vi "SetVariables.vi"(9 "Dynamic Runtime Property Vaslue":string, 10 "Dynamic Property Value":string, 11 "Sequence Context In":refnum<k7>) -> (0 "error out":errorcluster)   [LabVIEW 2011]
doc: "This VI demonstrates how to cast a SequenceFile object in order access properties of the PropertyObjectFile and PropertyObject parent classes"
uses:
  <vilib>/addons/TestStand/_TSUtility.llb/TestStand - Set Property Value (String).vi
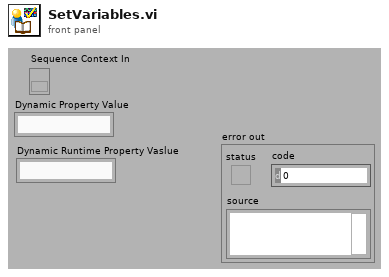
[diagram p1: front panel]
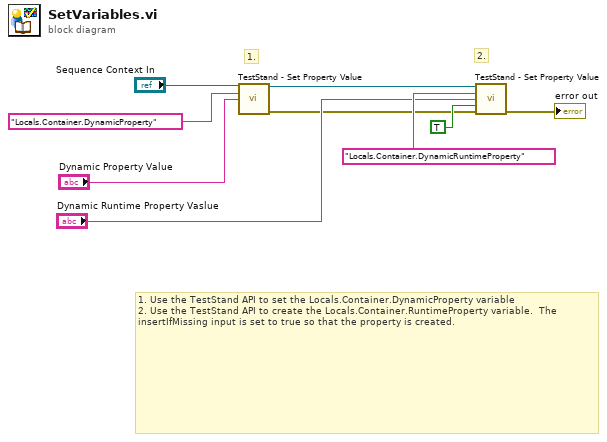
[diagram p0: block diagram]
diagram:
  # "2."
  # "1."
  # "1. Use the TestStand API to set the Locals.Container.DynamicProperty variable\n2. Use the TestStand API to create the Locals.Container.RuntimeProperty variable.  The insertIfMissing input is set to true so that the property is created."
  n1 = call-poly <vilib>:"TestStand - Set Property Value.vi"("Sequence Context In"="Sequence Context In", "Lookup String"="Locals.Container.DynamicProperty", "New Value"="Dynamic Property Value") -> ("Sequence Context Out"=w2:refnum<k7>, "error out"=w3:errorcluster)  [unwired: 11 in]
  n2 = call-poly <vilib>:"TestStand - Set Property Value.vi"("Sequence Context In"=w2, "Lookup String"="Locals.Container.DynamicRuntimeProperty", "New Value"="Dynamic Runtime Property Vaslue", "Insert If Missing"=TRUE, "error in (no error)"=w3) -> ("error out"=→"error out":errorcluster)  [unwired: 9 in, 1 out]
